vi "get last error.vi"(8 "error in (no error)":errorcluster, 10 "strbuffer_len":u64, 11 "error_out":string) -> (0 "error out":errorcluster, 2 "function return":u32(ring), 3 "error_out out":string)   [LabVIEW 2023, in "uhd.lvlib"]
doc: "UHD_API uhd_error uhd_get_last_error(char* error_out, size_t strbuffer_len);"
uses:
  <userlib>/uhd/uhd.lvlib
  <userlib>/uhd/uhd.dll
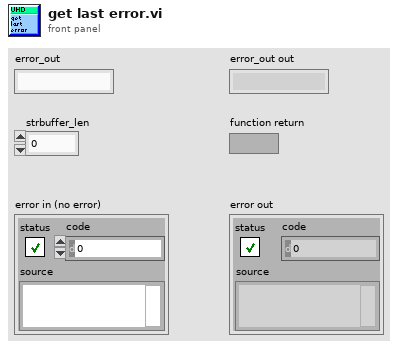
[diagram p1: front panel]
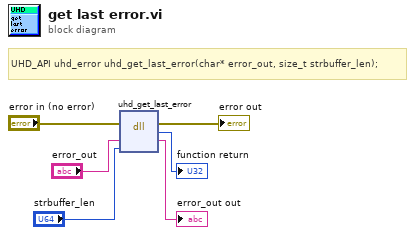
[diagram p0: block diagram]
diagram:
  # "UHD_API uhd_error uhd_get_last_error(char* error_out, size_t strbuffer_len);"
  n1 = dll-call lib="C:/Program Files/National Instruments/LabVIEW 2023/user.lib/uhd/uhd.*" fn="uhd_get_last_error"(error in="error in (no error)", "error_out"="error_out", "strbuffer_len"="strbuffer_len") -> (error out=→"error out":errorcluster, →"function return":u32, "error_out"=→"error_out out":string)  [unwired: 3 in, 1 out]
